vi "calc_thickness.vi"() -> ()   [LabVIEW 2021]
uses:
  <vilib>/Analysis/1siggen.llb/Ramp Pattern by Delta.vi
  <vilib>/Utility/file.llb/Read Delimited Spreadsheet (DBL).vi
  <vilib>/gmath/NI_Gmath.lvlib
  <vilib>/Analysis/NI_AALBase.lvlib
panel:
  out "Factor de atenuación":dbl
  in  "Material":T1(ring)=enum."Plomo"
  in  "Espesor (mm)":dbl=1.3
  out "error out":errorcluster
  in  "Energía Haz Incidente (keV)":dbl
  out "Coeficientes":cluster{"yi":dbl[], "xi used":dbl[]}[](graph)
  in  "error in (no error)":errorcluster
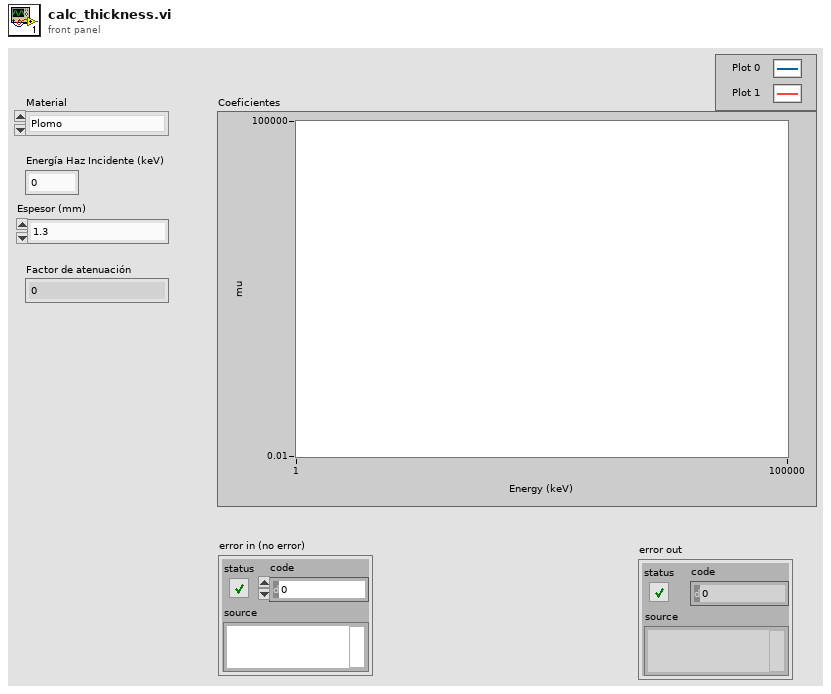
[diagram p1: front panel]
types:
  T1 = enum16{"Teflón", "Aluminio", "Agua", "Plomo", "Cobre"}
  T2 = cluster{"starting value":dbl, "increment":dbl, "final value":dbl}
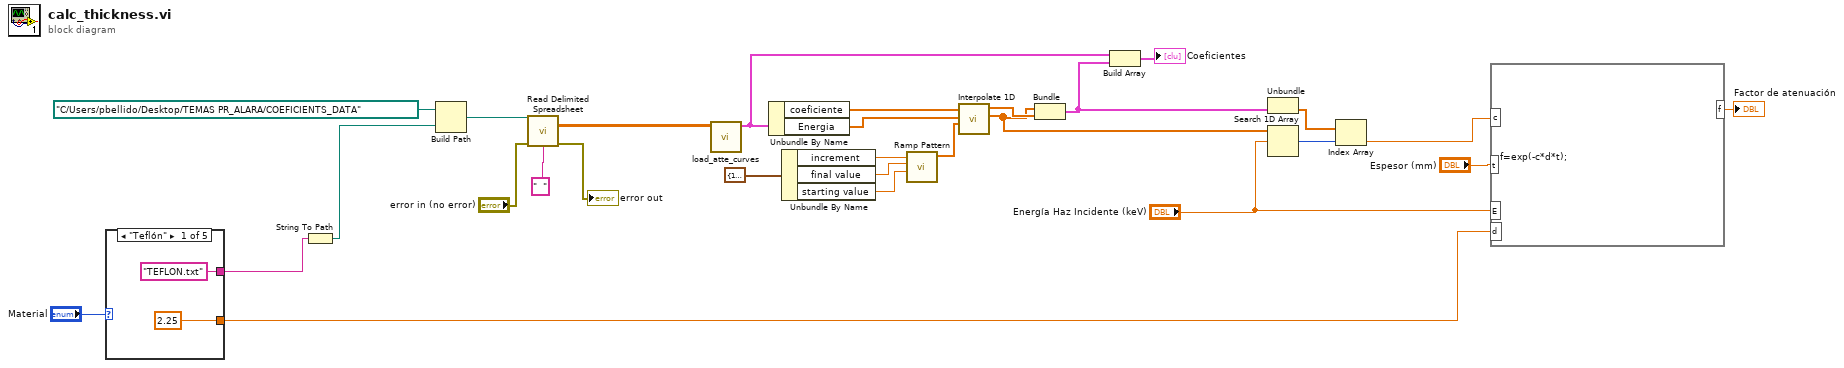
[diagram p0: block diagram]
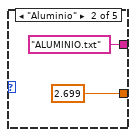
[diagram p2: hidden frame]
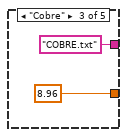
[diagram p3: hidden frame]
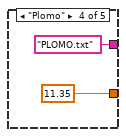
[diagram p4: hidden frame]
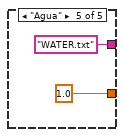
[diagram p5: hidden frame]
diagram:
  n1 = case shown="\"Teflón\"" "Material" {
    tunnel: [2.25 ("Densidad") 2.699 ("Densidad") 8.96 ("Densidad") 11.35 ("Densidad") 1.0 ("Densidad")] -> w7
    tunnel: ["TEFLON.txt" ("string") "ALUMINIO.txt" ("string") "COBRE.txt" ("string") "PLOMO.txt" ("string") "WATER.txt" ("string")] -> w1
    frame "Teflón" {
    }
    frame "Aluminio" {
    }
    frame "Cobre" {
    }
    frame "Plomo" {
    }
    frame "Agua" {
    }
  }
  n2 = String To Path(string=w1) -> (path=w2:path)
  n3 = Build Path(base path=path "C:/Users/pbellido/Desktop/TEMAS PR_ALARA/COEFICIENTS_DATA" ("Ruta  para el agua"), name or relative path=w2) -> (appended path=w3:path)
  n4 = call-poly <vilib>:"Read Delimited Spreadsheet.vi"("file path (dialog if empty)"=w3, "error in (no error)"="error in (no error)", "delimiter (\\t)"="  " ("delimiter (\\t)")) -> ("all rows"=w26:dbl[][], "error out"=→"error out":errorcluster)  [unwired: 7 in, 4 out]
  n5 = call "load_atte_curves.vi"("all rows"=w26) -> ("curva atenuation"=w18:cluster{"Energia":dbl[], "coeficiente":dbl[]})  [unwired: 10 in]
  n6 = Unbundle By Name(w18) -> ("coeficiente"=w25:dbl[], "Energia"=w24:dbl[])
  n7 = Unbundle By Name(T2 {"starting value"=10.0, "increment"=1.0, "final value"=5000.0} ("generate params")) -> ("increment"=w20:dbl, "final value"=w21:dbl, "starting value"=w22:dbl)
  n8 = call-poly <vilib>:"Ramp Pattern.vi"("start"=w22, "end"=w21, "delta"=w20) -> ("Ramp Pattern"=w19:dbl[])  [unwired: 6 in, 2 out]
  n9 = call <vilib>:"Interpolate 1D.vi"("xi"=w19, "X"=w24, "Y"=w25) -> ("xi used"=w15:dbl[], "yi"=w16:dbl[])  [unwired: 6 in, 1 out]
  n10 = Bundle("xi used"=w15, "yi"=w16) -> (w13:cluster{"xi used":dbl[], "yi":dbl[]})  [unwired: 1 in]
  n11 = Build Array(w18, w13) -> (→"Coeficientes":cluster{"xi used":dbl[], "yi":dbl[]}[])
  n12 = Unbundle(w13) -> ("yi"=w12:dbl[])  [unwired: 1 out]
  n13 = Search 1D Array(1D array=w15, element="Energía Haz Incidente (keV)") -> (index of element=w14:i32)  [unwired: 1 in]
  n14 = Index Array(array=w12, index=w14) -> (element=w10:dbl)
  n15 = formula code="f=exp(-c*d*t);"("E"="Energía Haz Incidente (keV)", "c"=w10, "d"=w7, "t"="Espesor (mm)") -> ("f"=→"Factor de atenuación":dbl)
